vi "RMS.vi"   [LabVIEW 2018, in "NI_AALPro.lvlib"]
doc: "Computes the root mean square (rms) of the input sequence <B>X</B>."
uses:
  <vilib>/Analysis/NI_AALPro.lvlib
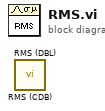
[diagram p0: block diagram]
diagram:
  n1 = call "RMS (CDB).vi"() -> ()  [unwired: 1 in, 2 out]
  n2 = call "RMS (DBL).vi"() -> ()  [unwired: 1 in, 2 out]
